vi "Update Index Array.vi"(4 "Y Dimension":i32, 6 "X Dimension":i32, 7 "Ribbon Mode":enum16{"Row", "Column"}(ring), 9 "Plot Range":T1, 10 "Index Array Input":u32[](array[numeric]), 11 "Ribbon Width":sgl) -> (1 "Point Offset":cluster{"X":sgl, "Y":sgl, "Z":sgl}, 2 "Index Array Output":u32[](array[numeric]))   [LabVIEW 2020, in "3D Ribbon.lvclass"]
uses:
  <vilib>/Math Plots/3D Math Plots/3D Ribbon/3D Ribbon/3D Ribbon.lvclass
  <vilib>/Math Plots/3D Math Plots/3D Plot/3D Plot/Typedef/Range Clusters.ctl
  <vilib>/Math Plots/3D Math Plots/3D Plot/3D Plot/3D Plot.lvclass
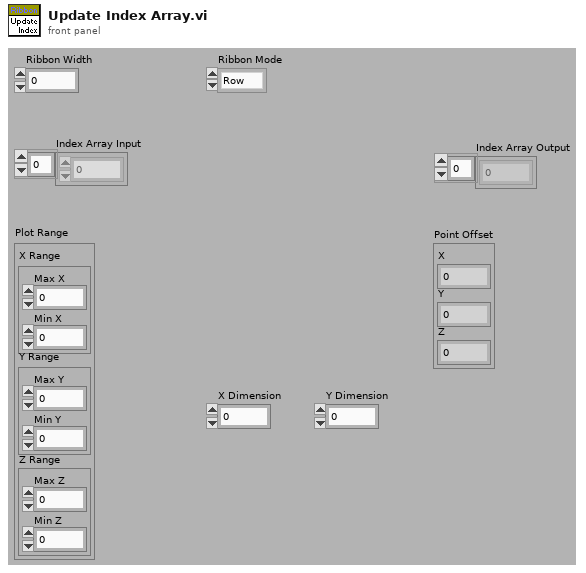
[diagram p1: front panel]
types:
  T1 = typedef "3D Plot.lvclass/Range Clusters.ctl" = cluster{"X Range":cluster{"Max X":sgl, "Min X":sgl}, "Y Range":cluster{"Max Y":sgl, "Min Y":sgl}, "Z Range":cluster{"Max Z":sgl, "Min Z":sgl}}
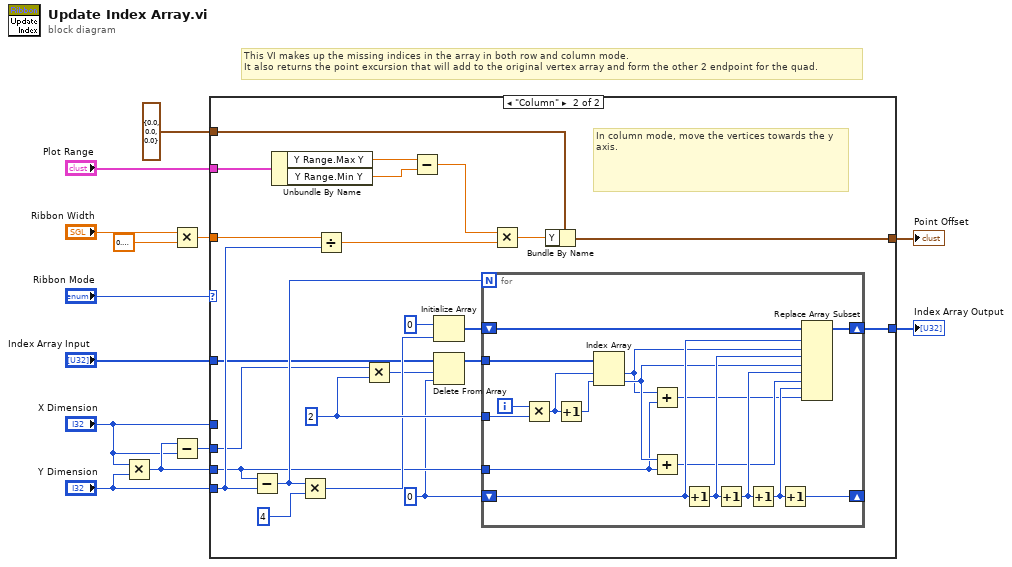
[diagram p0: block diagram]
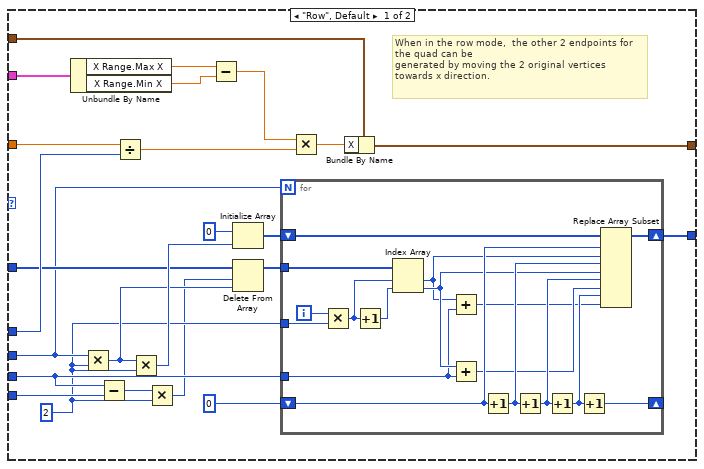
[diagram p2: hidden frame]
diagram:
  # "This VI makes up the missing indices in the array in both row and column mode.\nIt also returns the point excursion that will add to the original vertex array and form the other 2 endpoint for the quad."
  n1 = Multiply(x="X Dimension", y="Y Dimension") -> (x*y=w3:i32)
  n2 = Multiply(x="Ribbon Width", y=sgl 0.6) -> (x*y=w6:sgl)
  n3 = Subtract(x=w3, y="X Dimension") -> (x-y=w1:i32)
  n4 = case shown="\"Column\"" "Ribbon Mode" {
    tunnel: cluster{"X":sgl, "Y":sgl, "Z":sgl} {"X"=0.0, "Y"=0.0, "Z"=0.0} ("3D Point 2") -> [w37 w77]
    tunnel: w6 -> [w30 w76]
    tunnel: [w36 w75] -> w11
    tunnel: "Index Array Input" -> [w22 w58]
    tunnel: [w27 w67] -> w13
    tunnel: "X Dimension" -> [w23 _]
    tunnel: "Y Dimension" -> [w17 w64]
    tunnel: "Plot Range" -> [w35 w74]
    tunnel: w3 -> [w18 w61]
    tunnel: w1 -> [w19 w60]
    frame "Row", Default {
      w15 = 2 ("y")
      # "When in the row mode,  the other 2 endpoints for the quad can be\ngenerated by moving the 2 original vertices towards x direction."
      n5 = Unbundle By Name(w35) -> ("X Range.Max X"=w34:sgl, "X Range.Min X"=w33:sgl)
      n6 = Multiply(x=w19, y=w15) -> (x*y=w21:i32)
      n7 = Subtract(x=w18, y=w17) -> (x-y=w16:i32)
      n8 = Divide(x=w30, y=w23) -> (x/y=w29:sgl)
      n9 = Multiply(x=w21, y=w15) -> (x*y=w26:i32)
      n10 = Multiply(x=w16, y=w15) -> (x*y=w14:i32)
      n11 = Subtract(x=w34, y=w33) -> (x-y=w32:sgl)
      n12 = Initialize Array(u32 0, w26) -> (w24:u32[])
      n13 = Delete From Array(array=w22, length=w14, index=w21) -> (array with subset deleted=w20:u32[])  [unwired: 1 out]
      n14 = for {
        N: w19 -> [_]
        tunnel: w20 -> [w54]
        tunnel: w15 -> [w52]
        shift-right: [w49] -> _
        shift-left: 0 ("y") -> [w48]
        tunnel: w18 -> [w39]
        shift-right: [w42] -> w27
        shift-left: w24 -> [w41]
        i -> [w53]
        n15 = Multiply(x=w53, y=w52) -> (x*y=w51:i32)
        n16 = Increment(x=w51) -> (x+1=w50:i32)
        n17 = Index Array(array=w54, index #1=w51, index #2=w50) -> (element #1=w40:u32, element #2=w44:u32)
        n18 = Add(x=w40, y=w39) -> (x+y=w38:u32)
        n19 = Add(x=w44, y=w39) -> (x+y=w43:u32)
        n20 = Increment(x=w48) -> (x+1=w47:i32)
        n21 = Increment(x=w47) -> (x+1=w46:i32)
        n22 = Increment(x=w46) -> (x+1=w45:i32)
        n23 = Increment(x=w45) -> (x+1=w49:i32)
        n24 = Replace Array Subset(array=w41, new element #1=w40, index #1=w48, new element #2=w44, index #2=w47, new element #3=w43, index #3=w46, new element #4=w38, index #4=w45) -> (w42:u32[])
      }
      n25 = Multiply(x=w32, y=w29) -> (x*y=w31:sgl)
      n26 = Bundle By Name(cluster=w37, "X"=w31) -> (w36:cluster{"X":sgl, "Y":sgl, "Z":sgl})
    }
    frame "Column" {
      w55 = 0 ("y")
      w66 = 2 ("y")
      # "In column mode, move the vertices towards the y axis."
      n27 = Subtract(x=w61, y=w64) -> (x-y=w65:i32)
      n28 = Unbundle By Name(w74) -> ("Y Range.Max Y"=w73:sgl, "Y Range.Min Y"=w72:sgl)
      n29 = Multiply(x=w65, y=4) -> (x*y=w63:i32)
      n30 = Divide(x=w76, y=w64) -> (x/y=w69:sgl)
      n31 = Multiply(x=w60, y=w66) -> (x*y=w59:i32)
      n32 = Subtract(x=w73, y=w72) -> (x-y=w70:sgl)
      n33 = Initialize Array(u32 0, w63) -> (w68:u32[])
      n34 = Delete From Array(array=w58, length=w59, index=w55) -> (array with subset deleted=w57:u32[])  [unwired: 1 out]
      n35 = for {
        N: w65 -> [_]
        tunnel: w57 -> [w94]
        tunnel: w66 -> [w92]
        shift-right: [w89] -> _
        shift-left: w55 -> [w88]
        tunnel: w61 -> [w79]
        shift-right: [w82] -> w67
        shift-left: w68 -> [w81]
        i -> [w93]
        n36 = Multiply(x=w93, y=w92) -> (x*y=w91:i32)
        n37 = Increment(x=w91) -> (x+1=w90:i32)
        n38 = Index Array(array=w94, index #1=w91, index #2=w90) -> (element #1=w80:u32, element #2=w84:u32)
        n39 = Add(x=w80, y=w79) -> (x+y=w78:u32)
        n40 = Add(x=w84, y=w79) -> (x+y=w83:u32)
        n41 = Increment(x=w88) -> (x+1=w87:i32)
        n42 = Increment(x=w87) -> (x+1=w86:i32)
        n43 = Increment(x=w86) -> (x+1=w85:i32)
        n44 = Increment(x=w85) -> (x+1=w89:i32)
        n45 = Replace Array Subset(array=w81, new element #1=w80, index #1=w88, new element #2=w84, index #2=w87, new element #3=w83, index #3=w86, new element #4=w78, index #4=w85) -> (w82:u32[])
      }
      n46 = Multiply(x=w70, y=w69) -> (x*y=w71:sgl)
      n47 = Bundle By Name(cluster=w77, "Y"=w71) -> (w75:cluster{"X":sgl, "Y":sgl, "Z":sgl})
    }
  }
  "Index Array Output" <- w13
  "Point Offset" <- w11
